vi "Create All Message Queues.vi"(8 "error in (no error)":errorcluster) -> (0 "error out":errorcluster, 2 "PL Queues Array":refnum<queue>[](array[refnum]), 3 "All Message Queues out":T1)   [LabVIEW 2019, in "Message Queue.lvlib"]
doc: "This VI creates and initializes all the message queues for your application. If your application requires more than one message queue, right-click the \"Message Queues\" constant above and select Open Type Def. Add the new Message Queue(s) to the type definition, then initialize them in this VI."
uses:
  Message Queue.lvlib
  All Message Queues.ctl
  Message Cluster.ctl
  Enqueue Message (Single).vi
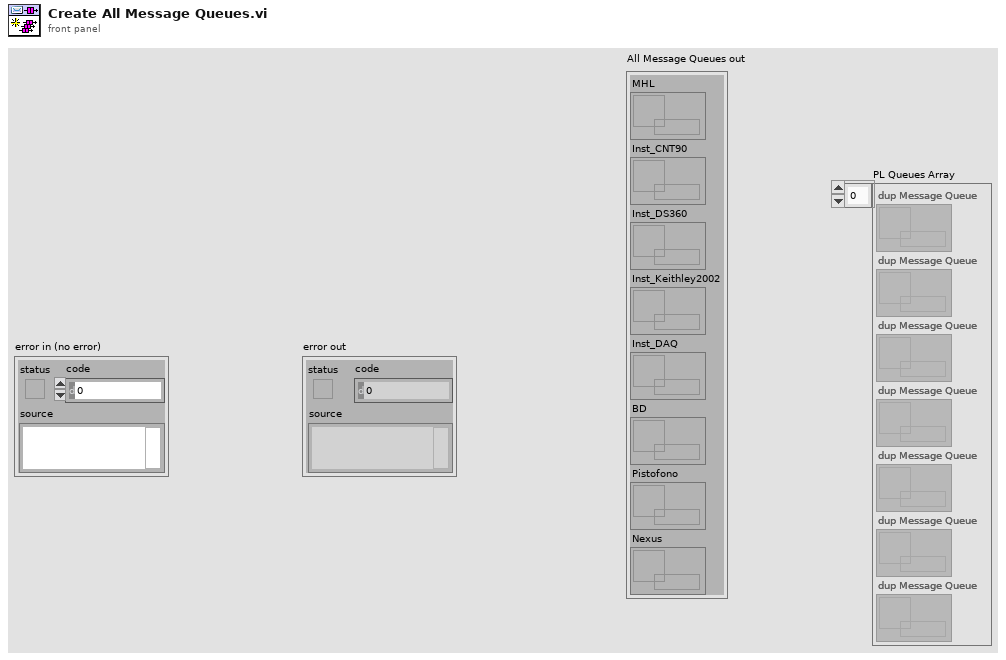
[diagram p1: front panel]
types:
  T1 = typedef "Message Queue.lvlib/All Message Queues.ctl" = cluster{"MHL":refnum<queue>, "Inst_CNT90":refnum<queue>, "Inst_DS360":refnum<queue>, "Inst_Keithley2002":refnum<queue>, "Inst_DAQ":refnum<queue>, "BD":refnum<queue>, "Pistofono":refnum<queue>, "Nexus":refnum<queue>}
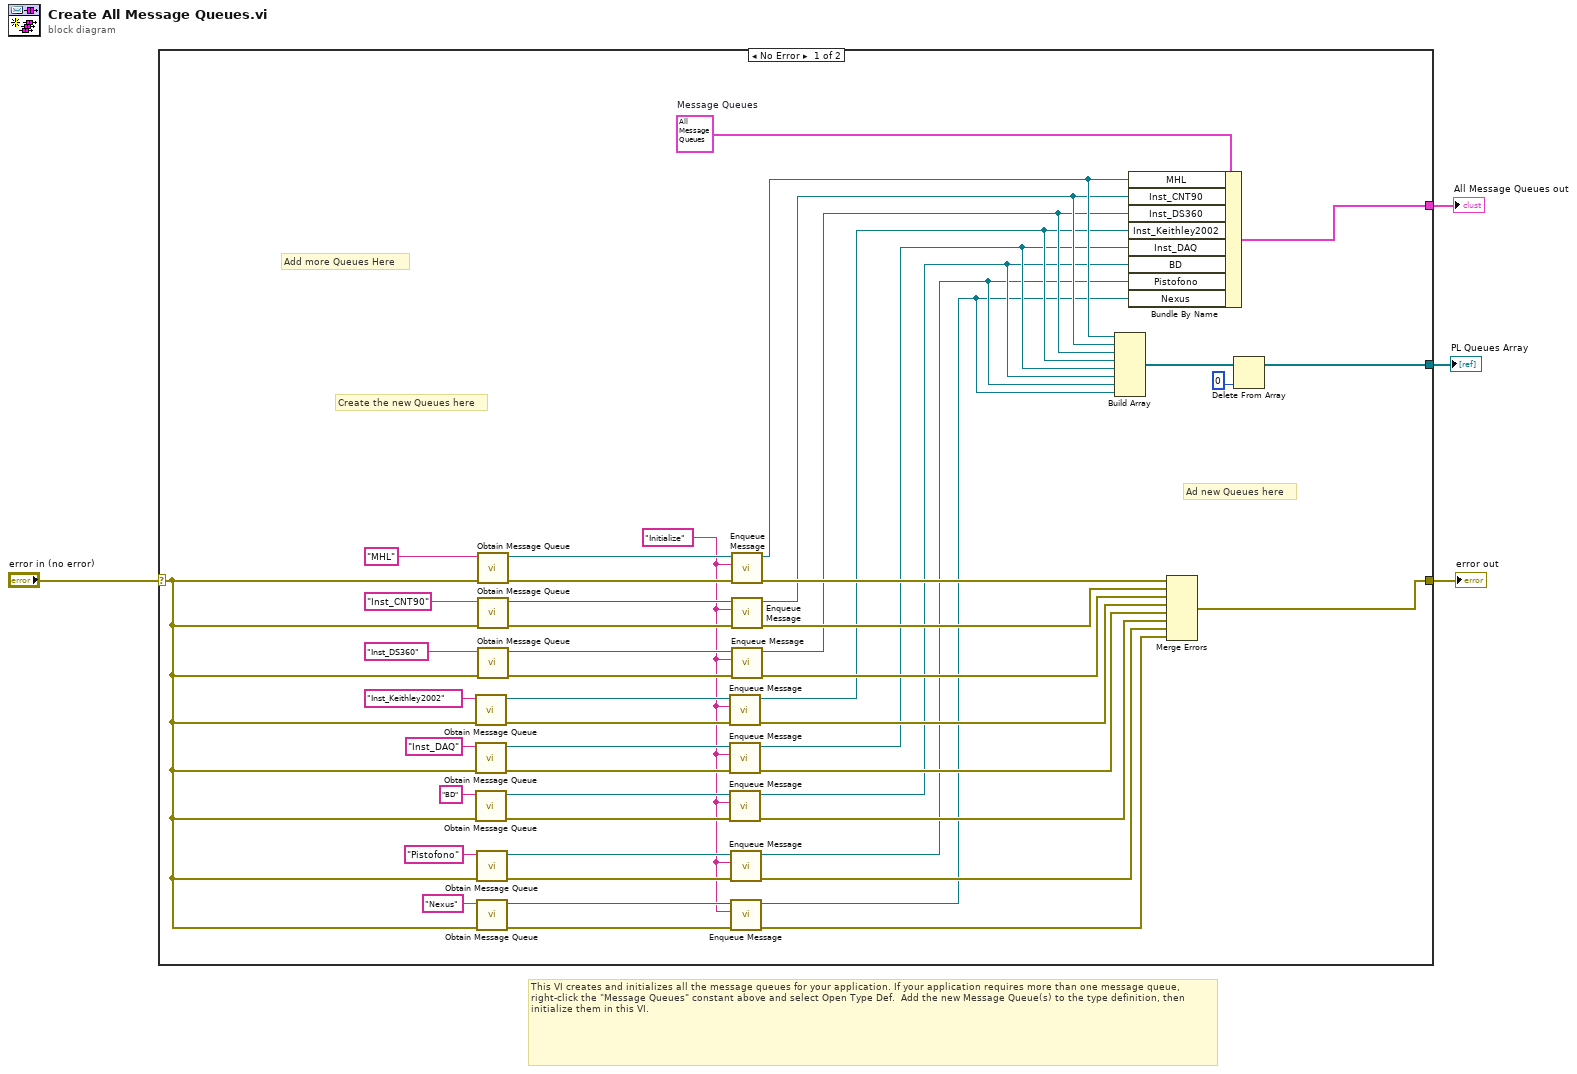
[diagram p0: block diagram]
diagram:
  # "This VI creates and initializes all the message queues for your application. If your application requires more than one message queue, right-click the \"Message Queues\" constant above and select Open Type Def.  Add the new Message Queue(s) to the type definition, then initialize them in this VI."
  n1 = case shown="No Error" "error in (no error)" {
    selector: "error in (no error)" -> [w8 w53]
    tunnel: [w41 w53] -> w4
    tunnel: [w51 _] -> w2
    tunnel: [w32 _] -> w1
    frame No Error {
      w5 = "Initialize" ("Message")
      w52 = T1 {"MHL"=refnum, "Inst_CNT90"=refnum, "Inst_DS360"=refnum, "Inst_Keithley2002"=refnum, "Inst_DAQ"=refnum, "BD"=refnum, "Pistofono"=refnum, "Nexus"=refnum}  # Message Queues
      # "Ad new Queues here"
      # "Create the new Queues here"
      # "Add more Queues Here"
      n2 = call "Obtain Message Queue.vi"("error in (no error)"=w8, "name (unnamed)"="Inst_Keithley2002") -> ("error out"=w46:errorcluster, "Message Queue"=w43:refnum<queue>)  [unwired: 8 in]
      n3 = call "Obtain Message Queue.vi"("error in (no error)"=w8, "name (unnamed)"="Inst_DAQ") -> ("error out"=w24:errorcluster, "Message Queue"=w25:refnum<queue>)  [unwired: 8 in]
      n4 = call "Obtain Message Queue.vi"("error in (no error)"=w8, "name (unnamed)"="BD") -> ("error out"=w19:errorcluster, "Message Queue"=w18:refnum<queue>)  [unwired: 8 in]
      n5 = call "Obtain Message Queue.vi"("error in (no error)"=w8, "name (unnamed)"="Pistofono") -> ("error out"=w14:errorcluster, "Message Queue"=w15:refnum<queue>)  [unwired: 8 in]
      n6 = call "Obtain Message Queue.vi"("error in (no error)"=w8, "name (unnamed)"="Nexus") -> ("error out"=w11:errorcluster, "Message Queue"=w10:refnum<queue>)  [unwired: 8 in]
      n7 = call "Obtain Message Queue.vi"("error in (no error)"=w8, "name (unnamed)"="MHL") -> ("error out"=w50:errorcluster, "Message Queue"=w49:refnum<queue>)  [unwired: 8 in]
      n8 = call "Obtain Message Queue.vi"("error in (no error)"=w8, "name (unnamed)"="Inst_CNT90") -> ("error out"=w48:errorcluster, "Message Queue"=w45:refnum<queue>)  [unwired: 8 in]
      n9 = call "Obtain Message Queue.vi"("error in (no error)"=w8, "name (unnamed)"="Inst_DS360") -> ("error out"=w47:errorcluster, "Message Queue"=w44:refnum<queue>)  [unwired: 8 in]
      n10 = call-poly "Enqueue Message.vi"("error in (no error)"=w46, "Message"=w5, "Message Queue"=w43) -> ("error out"=w38:errorcluster, "dup Message Queue"=w34:refnum<queue>)  [unwired: 7 in]
      n11 = call-poly "Enqueue Message.vi"("error in (no error)"=w24, "Message"=w5, "Message Queue"=w25) -> ("error out"=w22:errorcluster, "dup Message Queue"=w23:refnum<queue>)  [unwired: 7 in]
      n12 = call-poly "Enqueue Message.vi"("error in (no error)"=w19, "Message"=w5, "Message Queue"=w18) -> ("error out"=w21:errorcluster, "dup Message Queue"=w20:refnum<queue>)  [unwired: 7 in]
      n13 = call-poly "Enqueue Message.vi"("error in (no error)"=w14, "Message"=w5, "Message Queue"=w15) -> ("error out"=w13:errorcluster, "dup Message Queue"=w12:refnum<queue>)  [unwired: 7 in]
      n14 = call-poly "Enqueue Message.vi"("error in (no error)"=w11, "Message"=w5, "Message Queue"=w10) -> ("error out"=w7:errorcluster, "dup Message Queue"=w6:refnum<queue>)  [unwired: 7 in]
      n15 = call-poly "Enqueue Message.vi"("error in (no error)"=w50, "Message"=w5, "Message Queue"=w49) -> ("error out"=w42:errorcluster, "dup Message Queue"=w37:refnum<queue>)  [unwired: 7 in]
      n16 = call-poly "Enqueue Message.vi"("error in (no error)"=w48, "Message"=w5, "Message Queue"=w45) -> ("error out"=w40:errorcluster, "dup Message Queue"=w36:refnum<queue>)  [unwired: 7 in]
      n17 = call-poly "Enqueue Message.vi"("error in (no error)"=w47, "Message"=w5, "Message Queue"=w44) -> ("error out"=w39:errorcluster, "dup Message Queue"=w35:refnum<queue>)  [unwired: 7 in]
      n18 = Build Array(w37, w36, w35, w34, w23, w20, w12, w6) -> (w33:refnum<queue>[])
      n19 = Bundle By Name(cluster=w52, "MHL"=w37, "Inst_CNT90"=w36, "Inst_DS360"=w35, "Inst_Keithley2002"=w34, "Inst_DAQ"=w23, "BD"=w20, "Pistofono"=w12, "Nexus"=w6) -> (w51:T1)
      n20 = Merge Errors(w42, w40, w39, w38, w22, w21, w13, w7) -> (w41:errorcluster)
      n21 = Delete From Array(array=w33, index=0) -> (array with subset deleted=w32:refnum<queue>[])  [unwired: 1 in, 1 out]
    }
    frame Error {
    }
  }
  "All Message Queues out" <- w2
  "error out" <- w4
  "PL Queues Array" <- w1
